vi "Create Oneof Message Converters.vi"(8 "error in (no error)":errorcluster, 10 "Message parameters":T1[](array[typedef]), 11 "Library in":refnum<vi>) -> (0 "error out":errorcluster, 3 "Library out":refnum<vi>)   [LabVIEW 2019, in "gRPC Template Creation Utility.lvlib"]
uses:
  gRPC Template Creation Utility.lvlib
  TypeDefs/Message Metadata (Scripting).ctl
  TypeDefs/Message Element Metadata (Scripting).ctl
  TypeDefs/Message Element Type.ctl
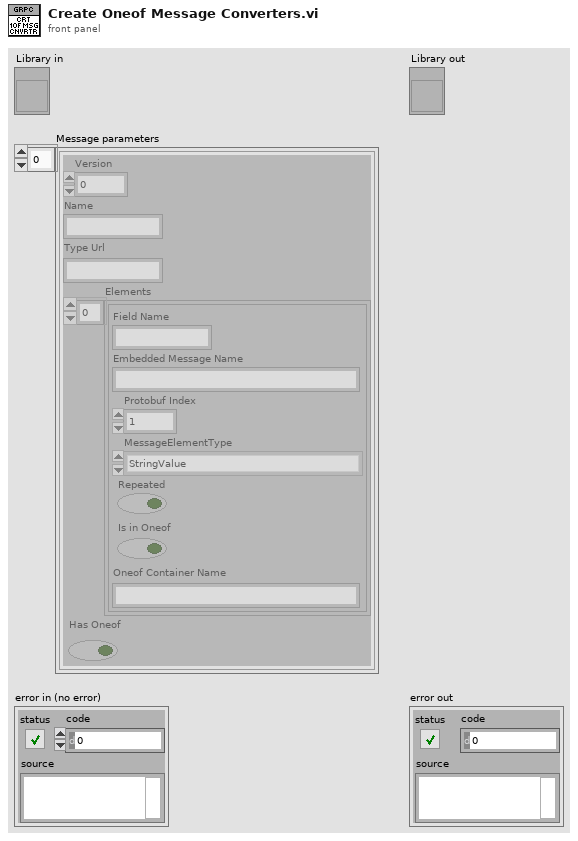
[diagram p1: front panel]
types:
  T1 = typedef "gRPC Template Creation Utility.lvlib/Message Metadata (Scripting).ctl" = cluster{"Version":i32, "Name":string, "Type Url":string, "Elements":T2[], "Has Oneof":bool}
  T2 = typedef "gRPC Template Creation Utility.lvlib/Message Element Metadata (Scripting).ctl" = cluster{"Field Name":string, "Embedded Message Name":string, "Protobuf Index":i32, "MessageElementType":T3, "Repeated":bool, "Is in Oneof":bool, "Oneof Container Name":string}
  T3 = typedef "gRPC Template Creation Utility.lvlib/Message Element Type.ctl" = enum32{"Int32Value", "FloatValue", "DoubleValue", "BoolValue", "StringValue", "MessageValue", "Int64Value", "UInt32Value", "UInt64Value", "EnumValue", "Bytes", "Fixed64", "Fixed32", "SFixed64", "SFixed32", "SInt64", "SInt32"}
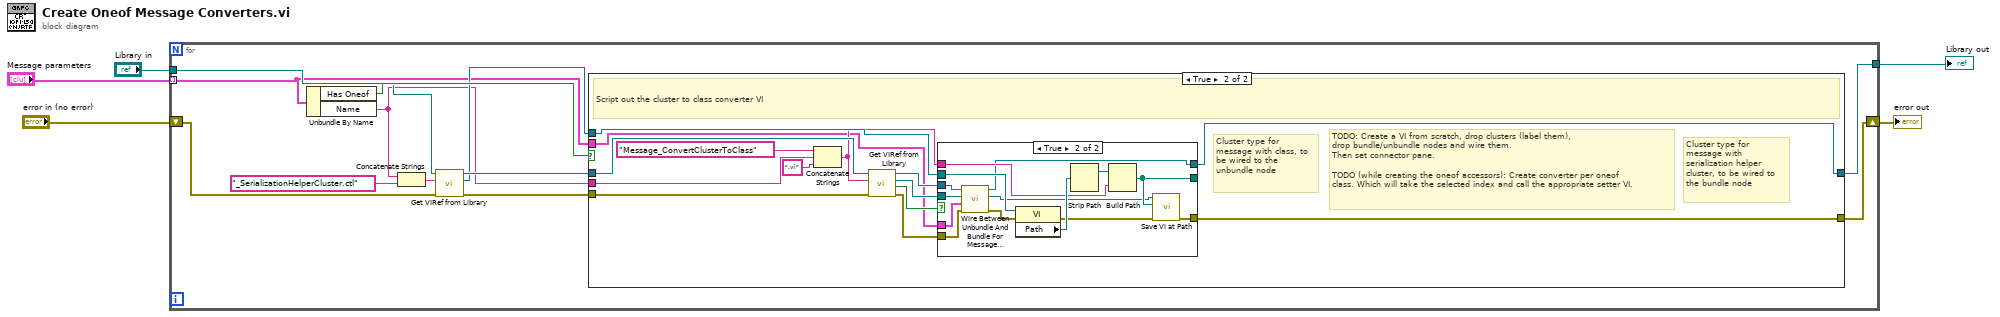
[diagram p0: block diagram]
diagram:
  n1 = for {
    tunnel: "Message parameters" -> [w6] mode=indexing
    shift-right: [w9] -> w3
    shift-left: "error in (no error)" -> [w12]
    tunnel: "Library in" -> [w16]
    tunnel: [w10] -> w5
    n2 = Unbundle By Name(w6) -> ("Has Oneof"=w17:bool, "Name"=w8:string)
    n3 = Concatenate Strings(w8, "_SerializationHelperCluster.ctl" ("string")) -> (w7:string)
    n4 = call "Get VIRef from Library.vi"("error in (no error)"=w12, "Item Name"=w7, "Library"=w16) -> ("error out"=w11:errorcluster, "VIref out"=w13:refnum<vi>, "Library"=w14:refnum<vi>)  [unwired: 5 in, 1 out]
    n5 = case shown="True" w17 {
      tunnel: w14 -> [w18 w26]
      tunnel: [w18 w28] -> w10
      tunnel: w13 -> [_ w32]
      tunnel: [_ w27] -> w9
      tunnel: w11 -> [_ w21]
      tunnel: w8 -> [_ w30]
      tunnel: w6 -> [_ w19]
      frame False {
      }
      frame True {
        # "TODO: Create a VI from scratch, drop clusters (label them),\ndrop bundle/unbundle nodes and wire them.\nThen set connector pane.\n\nTODO (while creating the oneof accessors): Create converter per oneof\nclass. Which will take the selected index and call the appropriate setter VI."
        # "Cluster type for message with serialization helper cluster, to be wired to the bundle node"
        # "Cluster type for message with class, to be wired to the unbundle node"
        # "Script out the cluster to class converter VI"
        n6 = Concatenate Strings("Message_ConvertClusterToClass", w30, ".vi" ("string")) -> (w25:string)
        n7 = call "Get VIRef from Library.vi"("error in (no error)"=w21, "Item Name"=w25, "Library"=w26) -> ("error out"=w20:errorcluster, "Found ?"=w23:bool, "VIref out"=w24:refnum<vi>, "Library"=w22:refnum<vi>)  [unwired: 5 in]
        n8 = case shown="True" w23 {
          tunnel: w32 -> [_ w48]
          tunnel: w20 -> [w34 w43]
          tunnel: [w33 w39] -> w28
          tunnel: [_ w42] -> _
          tunnel: [w34 w41] -> w27
          tunnel: w25 -> [_ w40]
          tunnel: w24 -> [_ w36]
          tunnel: w22 -> [w33 w37]
          tunnel: w19 -> [_ w35]
          frame False {
          }
          frame True {
            n9 = call "Wire Between Unbundle And Bundle For Message Converter With Oneof.vi"("error in (no error)"=w43, "Message Metadata"=w35, "VI Refnum"=w36, "Library ref in"=w37) -> ("error IO"=w45:errorcluster, "VI Refnum out"=w38:refnum<vi>, "Library ref out"=w39:refnum<vi>)  [unwired: 5 in]
            n10 = property class="VI"(reference=w48, error in=w45) -> (error out=w44:errorcluster, "Path"=w47:path)  [unwired: 1 out]
            n11 = Strip Path(path=w47) -> (stripped path=w46:path)  [unwired: 1 out]
            n12 = Build Path(base path=w46, name or relative path=w40) -> (appended path=w42:path)
            n13 = call "Save VI at Path.vi"("error in (no error)"=w44, "Path"=w42, "VI in"=w38) -> ("error out"=w41:errorcluster)  [unwired: 6 in, 2 out]
          }
        }
      }
    }
  }
  "Library out" <- w5
  "error out" <- w3
